vi "TARGET.vi"() -> ()   [LabVIEW 2018]
uses:
  <vilib>/Platform/TimedLoop/XDataNode/timing_clust.ctl
  <vilib>/Platform/TimedLoop/XDataNode/nitl_modes.ctl
  <vilib>/Platform/TimedLoop/XDataNode/wakeup.ctl
  <vilib>/rvi/eio/common/nirviEmuTemplateMethod_errors.vi
  <vilib>/rvi/Emulation/niFpgaGetClockAttributes.vi
  <vilib>/rvi/Emulation/niFpgaSctlEmulationGetInTimedLoop.vi
  <vilib>/rvi/Emulation/niFpgaEmulationReportErrorSimple.vi
  <vilib>/rvi/Emulation/niFpgaCriticalErrorInLSC.vi
  <vilib>/rvi/Memory/Memory_Emulation/niFpgaMemoryFastEmulationDramWriteAndRequestData.vi
  <vilib>/rvi/Memory/Memory_Emulation/niFpgaMemoryEmulationDramWriteAndRequestData.vi
  <vilib>/rvi/DataTransferAndStorage/Container/Common/niFpgaContainerGetUniqueNameForEmu.vi
  <vilib>/rvi/Memory/Memory_Emulation/niFpgaMemoryEmulationDramWriteAndRequestDataApplyByteEnables.vi
  <vilib>/rvi/DataTransferAndStorage/Container/Common/niFpgaContainerExecOnDevCompGetState.vi
  <vilib>/rvi/Emulation/niFpgaProcessEmulError.vi
  <vilib>/rvi/interface/RandomDataEmulation/niFpgaRandomDataHandleErrors.vi
  <vilib>/eio/EIONode/EIONode.xnode
  <vilib>/Platform/TimedLoop/XDataNode/XDataNode.xnode
  <vilib>/rvi/DataTransferAndStorage/Container/XNode/niFpgaContainer.xnode
  <vilib>/rvi/Memory/Memory_Emulation/niFpgaMemoryEmulationDramRetrieveDataRefIn.vi
  <vilib>/rvi/interface/RandomDataEmulation/nirviRandomDataFpgaReadWriteTemplate.vi
  <vilib>/Platform/TimedLoop/XDataNode/XDNodeRunTimeDep.lvlib
panel:
  in  "RESET":bool
  in  "ENABLE":bool
  in  "BI":bool
  in  "SERADD":bool
  out "Фронты":u16
  in  "65535":u16=65535
  in  "Температура?":bool
  in  "Кон.адр.":u32=47804
  in  "39":u16=39
  in  "30":u16=30
  in  "20":u16=20
  in  "39":u16=39
  in  "1332":u16=1332
  in  "40":u16=40
  in  "1036":u16=1036
  in  "1550":u16=1550
  in  "Линейки":bool
  in  "Запись":bool
  in  "Нач.адр.":u32
  out "DATA":bool[](array[boolean])
  in  "I2C[37:0]_READ":bool[](array[boolean])=[FALSE, FALSE, FALSE, FALSE, FALSE, FALSE, FALSE, FALSE, FALSE, FALSE, FALSE, FALSE, FALSE, FALSE, FALSE, FALSE, FALSE, FALSE, FALSE, FALSE, FALSE, FALSE, FALSE, FALSE, FALSE, FALSE, FALSE, FALSE, FALSE, FALSE, FALSE, FALSE, FALSE, FALSE, FALSE, FALSE, FALSE, FALSE]
  in  "I2C[26:0]_WRITE":bool[](array[boolean])=[FALSE, FALSE, FALSE, FALSE, FALSE, FALSE, FALSE, FALSE, FALSE, FALSE, FALSE, FALSE, FALSE, FALSE, FALSE, FALSE, FALSE, FALSE, FALSE, FALSE, FALSE, FALSE, FALSE, FALSE, FALSE, FALSE, FALSE]
  in  "R(T)/W(F)":bool
  in  "Регистр!":bool
  in  "Остановка основого цикла":bool
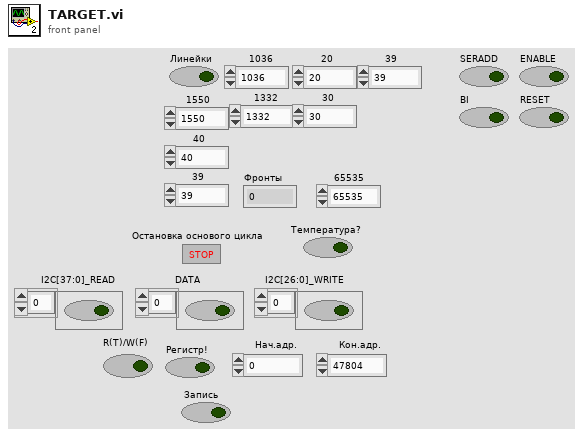
[diagram p1: front panel]
types:
  T1 = typedef "XDNodeRunTimeDep.lvlib/timing_clust.ctl" = cluster{"Expected End [f-1]":u64, "Actual End [f-1]":u64, "Finished Late? [f-1]":bool, "Expected End [i-1]":u64, "Actual End [i-1]":u64, "Finished Late? [i-1]":bool, "Expected Start [i]":u64, "Actual Start [i]":u64, "Expected Start [f]":u64, "Actual Start [f]":u64, "Source Name":string, "Structure Name":string, "Period":i64, "Deadline":i64, "Offset":i64, "Start":i64, "Priority":i32, "Timeout":i32, "Mode":T2, "Wakeup Reason":T3, "Error":errorcluster, "Source Type":string, "Secondary Source Type":string, "Global End Time":u64, "Global Start Time":u64, "Frame Duration":u64, "Iteration Duration":u64, "Assigned CPU":i32, "I/O Scan Engine Mode":u32}
  T2 = typedef "XDNodeRunTimeDep.lvlib/nitl_modes.ctl" = enum32{"No Change", "Process missed periods, maintain original phase", "Discard missed periods, maintain original phase", "Process missed periods, ignore original phase", "Discard missed periods, ignore original phase"}
  T3 = typedef "XDNodeRunTimeDep.lvlib/wakeup.ctl" = enum32{"Normal", "Aborted", "Asynchronous wakeup", "Timing source error", "Timed loop error", "Timeout"}
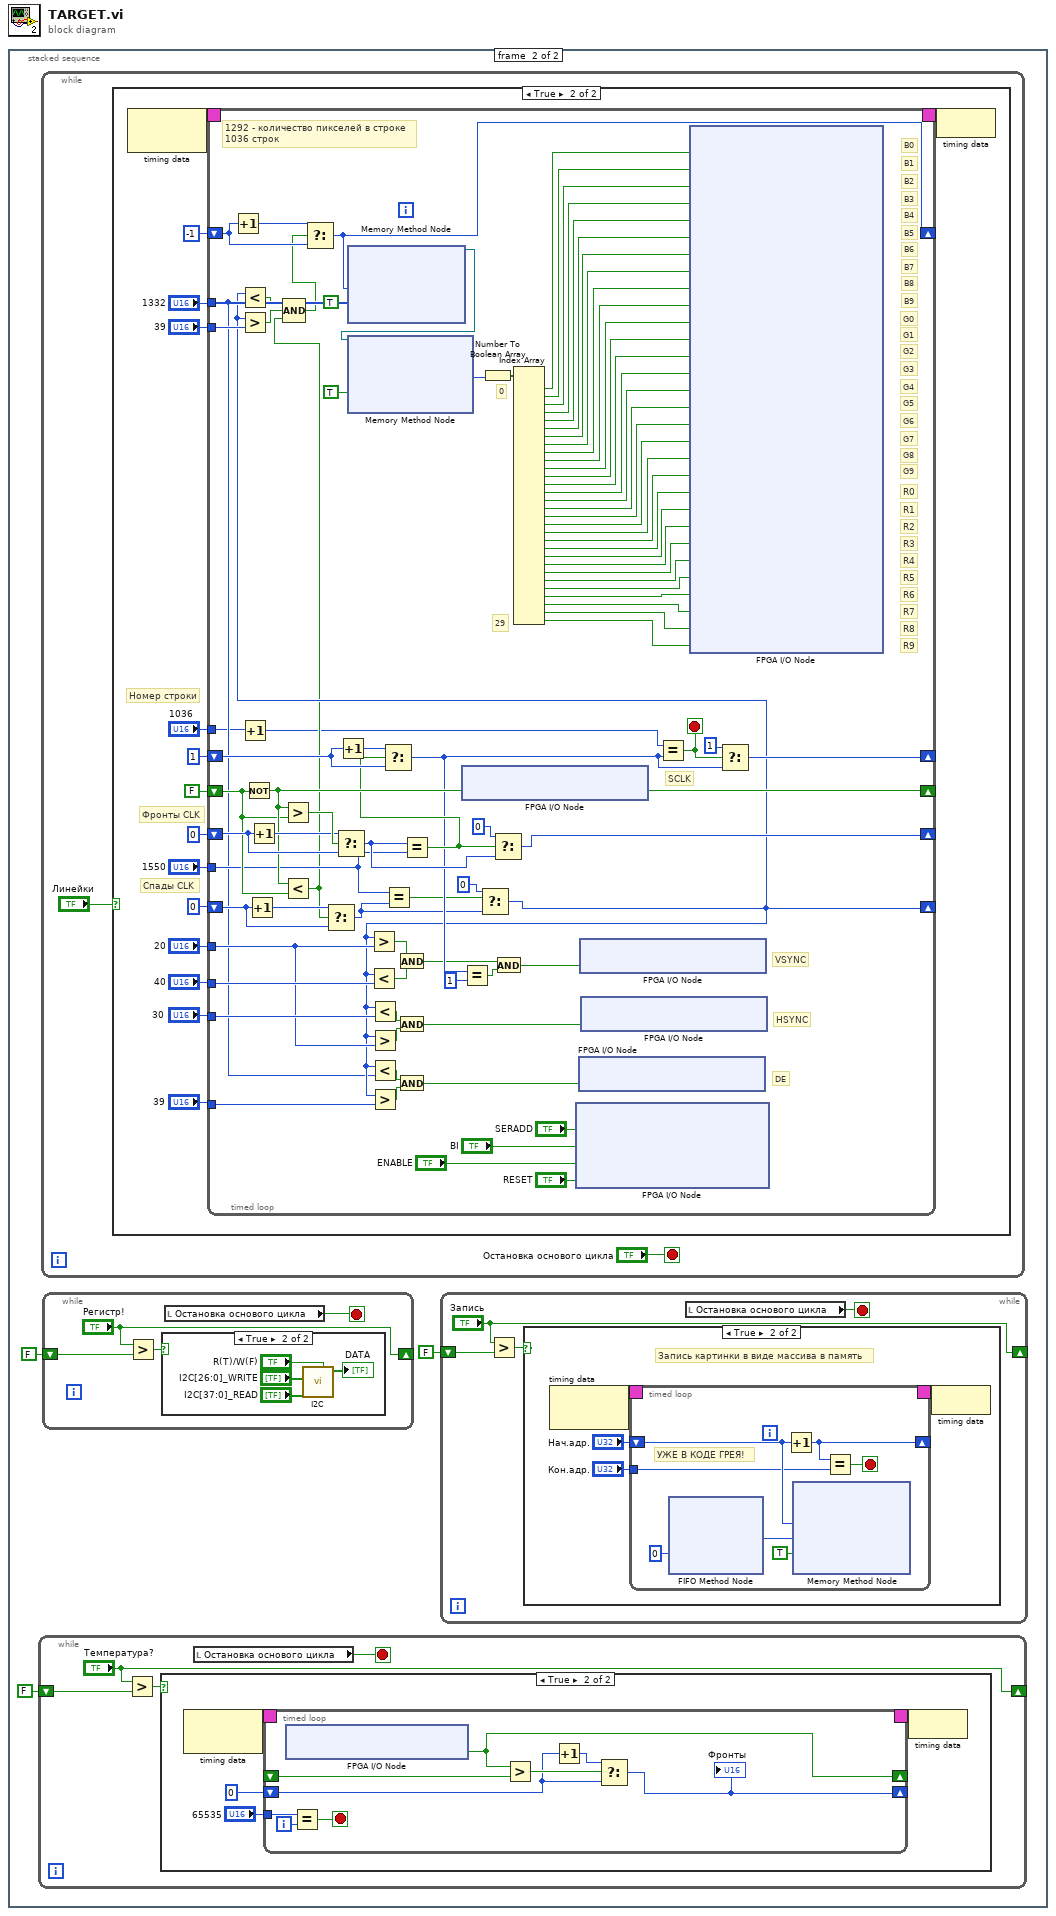
[diagram p0: block diagram]
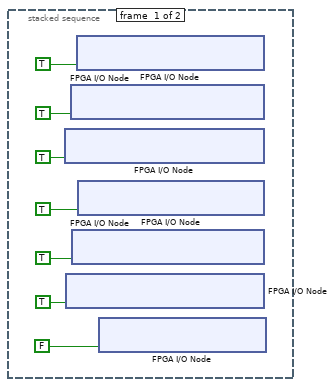
[diagram p2: hidden frame]
diagram:
  n1 = stacked-sequence {
    frame #0 {
      n2 = xnode "FPGA I/O Node"("IO Module\\DDCA_DIO16-23_WE"=TRUE) -> ()  [unwired: 1 in, 1 out]
      n3 = xnode "FPGA I/O Node"("IO Module\\DDCB_DIO16-23_WE"=TRUE) -> ()  [unwired: 1 in, 1 out]
      n4 = xnode "FPGA I/O Node"("IO Module\\DDCA_DIO8-15_WE"=TRUE) -> ()  [unwired: 1 in, 1 out]
      n5 = xnode "FPGA I/O Node"("IO Module\\DDCB_DIO8-15_WE"=TRUE) -> ()  [unwired: 1 in, 1 out]
      n6 = xnode "FPGA I/O Node"("IO Module\\DDCA_DIO0-7_WE"=TRUE) -> ()  [unwired: 1 in, 1 out]
      n7 = xnode "FPGA I/O Node"("IO Module\\DDCB_DIO0-7_WE"=TRUE) -> ()  [unwired: 1 in, 1 out]
      n8 = xnode "FPGA I/O Node"("IO Module\\DDCB_PFI_WE"=FALSE) -> ()  [unwired: 1 in, 1 out]
    }
    frame #1 {
      n9 = while {
        shift-right: ["Температура?"] -> _
        shift-left: FALSE ("Температура?") -> [w13]
        stop <- w14 stop-if-true
        n10 = Greater?(x="Температура?", y=w13) -> (0:w11:bool)
        n11 = case shown="True" w11 {
          frame False {
          }
          frame True {
            n12 = node-c288() -> (w18:T1)  [unwired: 1 in]
            n13 = timed-loop {
              timing: w18 -> [_]
              timing-out: [_] -> w17
              tunnel: "65535" -> [w25]
              shift-right: [w20] -> _
              shift-left: u16 0 -> [w21]
              shift-right: [w19] -> _
              shift-left: _ -> [w27]
              i -> [w26]
              stop <- w24 stop-if-true
              n14 = xnode "FPGA I/O Node"() -> ("IO Module\\DDCB_PFI1_Read"=w19:bool)  [unwired: 1 in, 1 out]
              n15 = Equal?(x=w25, y=w26) -> (x = y?=w24:bool)
              n16 = Greater?(x=w19, y=w27) -> (0:w23:bool)
              n17 = Increment(x=w21) -> (x+1=w22:u16)
              n18 = Select(t=w22, s=w23, f=w21) -> (s? t:f=w20:u16)
              "Фронты" <- w20
            }
            n19 = node-c288(w17) -> ()
          }
        }
        n20 = local read "Остановка основого цикла"() -> (w14:bool)
      }
      n21 = while {
        stop <- "Остановка основого цикла" stop-if-true
        n22 = case shown="True" "Линейки" {
          frame False {
          }
          frame True {
            # "Спады CLK"
            # "Фронты CLK"
            # "Номер строки"
            n23 = node-c288() -> (w75:T1)  [unwired: 1 in]
            n24 = timed-loop {
              timing: w75 -> [_]
              timing-out: [_] -> w74
              shift-right: [w146] -> _
              shift-left: u32 1 -> [w162]
              shift-right: [w158] -> _
              shift-left: FALSE -> [w157]
              shift-right: [w138] -> _
              shift-left: u16 0 -> [w159]
              shift-right: [w89] -> _
              shift-left: u16 0 -> [w155]
              tunnel: "1550" -> [w145]
              tunnel: "20" -> [w94]
              tunnel: "1036" -> [w81]
              tunnel: "40" -> [w137]
              shift-right: [w131] -> _
              shift-left: -1 -> [w132]
              tunnel: "1332" -> [w88]
              tunnel: "39" -> [w130]
              tunnel: "30" -> [w97]
              tunnel: "39" -> [w87]
              stop <- w149 stop-if-true
              # "B9"
              # "B8"
              # "B7"
              # "B6"
              # "B5"
              # "B4"
              # "B3"
              # "B2"
              # "B1"
              # "B0"
              # "29"
              # "0"
              # "1292 - количество пикселей в строке\n1036 строк"
              # "HSYNC"
              # "VSYNC"
              # "DE"
              # "SCLK"
              # "G9"
              # "G8"
              # "G7"
              # "G6"
              # "G5"
              # "G4"
              # "G3"
              # "G2"
              # "G1"
              # "G0"
              # "R9"
              # "R8"
              # "R7"
              # "R6"
              # "R5"
              # "R4"
              # "R3"
              # "R2"
              # "R1"
              # "R0"
              n25 = Increment(x=w132) -> (x+1=w133:i32)
              n26 = Increment(x=w81) -> (x+1=w80:u16)
              n27 = Not(x=w157) -> (.not. x?=w158:bool)
              n28 = Increment(x=w155) -> (x+1=w156:u16)
              n29 = Increment(x=w159) -> (x+1=w160:u16)
              n30 = Greater?(x=w158, y=w157) -> (0:w161:bool)
              n31 = Less?(x=w158, y=w157) -> (x < y?=w83:bool)
              n32 = Select(t=w156, s=w83, f=w155) -> (s? t:f=w142:u16)
              n33 = Select(t=w160, s=w161, f=w159) -> (s? t:f=w152:u16)
              n34 = Increment(x=w162) -> (x+1=w163:u32)
              n35 = Equal?(x=w145, y=w142) -> (x = y?=w144:bool)
              n36 = Equal?(x=w152, y=w145) -> (x = y?=w153:bool)
              n37 = Select(t=w163, s=w153, f=w162) -> (s? t:f=w147:u32)
              n38 = xnode "FPGA I/O Node"("IO Module\\DDCB_DIO4_Write"=w158) -> ()  [unwired: 1 in, 1 out]
              n39 = Equal?(x=w147, y=u32 1) -> (x = y?=w150:bool)
              n40 = Select(t=u16 0, s=w144, f=w142) -> (s? t:f=w89:u16)
              n41 = Less?(x=w89, y=w88) -> (x < y?=w85:bool)
              n42 = Greater?(x=w89, y=w130) -> (0:w84:bool)
              n43 = Compound Arithmetic op=AND(w85, w84, w83) -> (w82:bool)
              n44 = Select(t=w133, s=w82, f=w132) -> (s? t:f=w131:i32)
              n45 = xnode ("Memory Method Node")("Address"=w131, "Input Valid"=TRUE) -> ("Memory Out"=w141:refnum<k21>)  [unwired: 1 in, 1 out]
              n46 = xnode ("Memory Method Node")("Ready for Output"=TRUE ("Input Valid"), "Memory In"=w141) -> ("Data"=w129:u32)  [unwired: 2 out]
              n47 = Greater?(x=w89, y=w94) -> (0:w136:bool)
              n48 = Less?(x=w89, y=w137) -> (x < y?=w135:bool)
              n49 = Less?(x=w89, y=w97) -> (x < y?=w96:bool)
              n50 = Greater?(x=w89, y=w94) -> (0:w95:bool)
              n51 = Less?(x=w89, y=w88) -> (x < y?=w90:bool)
              n52 = Greater?(x=w89, y=w87) -> (0:w91:bool)
              n53 = And(x=w136, y=w135) -> (x .and. y?=w134:bool)
              n54 = And(x=w96, y=w95) -> (x .and. y?=w92:bool)
              n55 = And(x=w90, y=w91) -> (x .and. y?=w86:bool)
              n56 = Number To Boolean Array(number=w129) -> (Boolean array=w128:bool[])
              n57 = Select(t=u16 0, s=w153, f=w152) -> (s? t:f=w138:u16)
              n58 = And(x=w134, y=w150) -> (x .and. y?=w93:bool)
              n59 = Index Array(array=w128) -> (element #1=w127:bool, element #2=w126:bool, element #3=w125:bool, element #4=w124:bool, element #5=w123:bool, element #6=w122:bool, element #7=w121:bool, element #8=w120:bool, element #9=w119:bool, element #10=w118:bool, element #11=w117:bool, element #12=w116:bool, element #13=w115:bool, element #14=w114:bool, element #15=w113:bool, element #16=w112:bool, element #17=w111:bool, element #18=w110:bool, element #19=w109:bool, element #20=w108:bool, element #21=w107:bool, element #22=w106:bool, element #23=w105:bool, element #24=w104:bool, element #25=w103:bool, element #26=w102:bool, element #27=w101:bool, element #28=w100:bool, element #29=w99:bool, element #30=w98:bool)  [unwired: 30 in]
              n60 = xnode "FPGA I/O Node"("IO Module\\DDCA_DIO20_Write"="SERADD", "IO Module\\DDCB_DIO0_Write"="BI", "IO Module\\DDCB_DIO5_Write"="ENABLE", "IO Module\\DDCB_DIO6_Write"="RESET") -> ()  [unwired: 4 in, 4 out]
              n61 = xnode "FPGA I/O Node"("IO Module\\DDCB_DIO3_Write"=w86) -> ()  [unwired: 1 in, 1 out]
              n62 = xnode "FPGA I/O Node"("IO Module\\DDCB_DIO1_Write"=w93) -> ()  [unwired: 1 in, 1 out]
              n63 = xnode "FPGA I/O Node"("IO Module\\DDCB_DIO2_Write"=w92) -> ()  [unwired: 1 in, 1 out]
              n64 = Equal?(x=w80, y=w147) -> (x = y?=w149:bool)
              n65 = xnode "FPGA I/O Node"("IO Module\\DDCA_DIO9_Write"=w127, "IO Module\\DDCA_DIO8_Write"=w126, "IO Module\\DDCA_DIO7_Write"=w125, "IO Module\\DDCA_DIO6_Write"=w124, "IO Module\\DDCA_DIO5_Write"=w123, "IO Module\\DDCA_DIO4_Write"=w122, "IO Module\\DDCA_DIO3_Write"=w121, "IO Module\\DDCA_DIO2_Write"=w120, "IO Module\\DDCA_DIO1_Write"=w119, "IO Module\\DDCA_DIO0_Write"=w118, "IO Module\\DDCB_DIO16_Write"=w117, "IO Module\\DDCB_DIO15_Write"=w116, "IO Module\\DDCB_DIO14_Write"=w115, "IO Module\\DDCB_DIO13_Write"=w114, "IO Module\\DDCB_DIO12_Write"=w113, "IO Module\\DDCB_DIO11_Write"=w112, "IO Module\\DDCB_DIO10_Write"=w111, "IO Module\\DDCB_DIO9_Write"=w110, "IO Module\\DDCB_DIO8_Write"=w109, "IO Module\\DDCB_DIO7_Write"=w108, "IO Module\\DDCA_DIO19_Write"=w107, "IO Module\\DDCA_DIO18_Write"=w106, "IO Module\\DDCA_DIO17_Write"=w105, "IO Module\\DDCA_DIO16_Write"=w104, "IO Module\\DDCA_DIO15_Write"=w103, "IO Module\\DDCA_DIO14_Write"=w102, "IO Module\\DDCA_DIO13_Write"=w101, "IO Module\\DDCA_DIO12_Write"=w100, "IO Module\\DDCA_DIO11_Write"=w99, "IO Module\\DDCA_DIO10_Write"=w98) -> ()  [unwired: 30 in, 30 out]
              n66 = Select(t=u32 1, s=w149, f=w147) -> (s? t:f=w146:u32)
            }
            n67 = node-c288(w74) -> ()
          }
        }
      }
      n68 = while {
        shift-right: ["Регистр!"] -> _
        shift-left: FALSE ("Регистр!") -> [w54]
        stop <- w51 stop-if-true
        n69 = Greater?(x="Регистр!", y=w54) -> (0:w52:bool)
        n70 = case shown="True" w52 {
          frame False {
          }
          frame True {
            n71 = call "I2C.vi"("I2C[37:0]_READ"="I2C[37:0]_READ", "I2C[26:0]_WRITE"="I2C[26:0]_WRITE", "R(T)/W(F)"="R(T)/W(F)") -> ("DATA"=→"DATA":bool[])  [unwired: 8 in]
          }
        }
        n72 = local read "Остановка основого цикла"() -> (w51:bool)
      }
      n73 = while {
        shift-right: ["Запись"] -> _
        shift-left: FALSE ("Запись картинки в память") -> [w34]
        stop <- w35 stop-if-true
        n74 = Greater?(x="Запись", y=w34) -> (0:w32:bool)
        n75 = case shown="True" w32 {
          frame False {
          }
          frame True {
            # "Запись картинки в виде массива в память"
            n76 = node-c288() -> (w39:T1)  [unwired: 1 in]
            n77 = timed-loop {
              timing: w39 -> [_]
              timing-out: [_] -> w38
              shift-right: [w41] -> _
              shift-left: "Нач.адр." -> [w42]
              tunnel: "Кон.адр." -> [w40]
              stop <- w46 stop-if-true
              # "УЖЕ В КОДЕ ГРЕЯ!"
              n78 = xnode ("FIFO Method Node")("Timeout"=0) -> ("Element"=w45:u32)  [unwired: 1 in, 2 out]
              n79 = Increment(x=w42) -> (x+1=w41:u32)
              n80 = xnode ("Memory Method Node")("Address"=w42, "Data"=w45, "Input Valid"=TRUE) -> ()  [unwired: 1 in, 2 out]
              n81 = Equal?(x=w41, y=w40) -> (x = y?=w46:bool)
            }
            n82 = node-c288(w38) -> ()
          }
        }
        n83 = local read "Остановка основого цикла"() -> (w35:bool)
      }
    }
  }
